vi "Configure Integration Filter.vi"(8 "error in (no error)":errorcluster, 9 "Measurement Speed (1 PLC)":dbl=1.0 format="%.2g", 10 "Function (0: Volts)":u16(ring) items=["Volts", "Current", "Resistance"], 11 "VISA resource name":refnum<visa-resource-name>) -> (0 "error out":errorcluster, 3 "VISA resource name out":refnum<visa-resource-name>)   [LabVIEW 2017, in "Keithley 2450.lvlib"]
doc: "Configures the amount of time spent integrating the measurement before returning a measurement. This time is expressed in power line cycles."
uses:
  Keithley 2450.lvlib
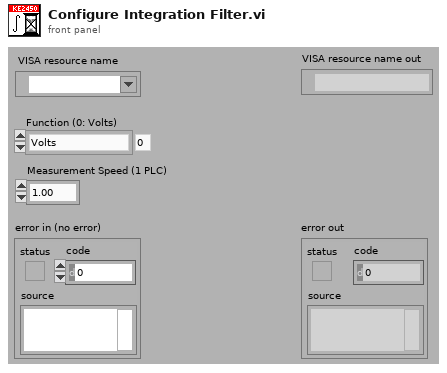
[diagram p1: front panel]
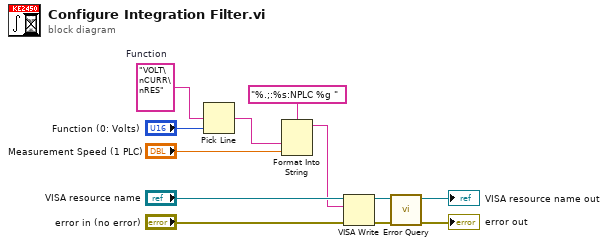
[diagram p0: block diagram]
diagram:
  w4 = "VOLT\nCURR\nRES"  # Function
  n1 = Pick Line(multi-line string=w4, line index="Function (0: Volts)") -> (output string=w1:string)  [unwired: 1 out]
  n2 = Format Into String(format string="%.;:%s:NPLC %g ", w1, "Measurement Speed (1 PLC)") -> (resulting string=w5:string)  [unwired: 2 in, 1 out]
  n3 = VISA Write(VISA resource name="VISA resource name", write buffer=w5, error in (no error)="error in (no error)") -> (VISA resource name out=w8:refnum<visa-resource-name>, error out=w7:errorcluster)  [unwired: 1 out]
  n4 = call "Error Query.vi"("error in (no error)"=w7, "VISA resource name"=w8) -> ("error out"=→"error out":errorcluster, "VISA resource name out"=→"VISA resource name out":refnum<visa-resource-name>)  [unwired: 8 out]
